vi "Constructor.vi"(8 "error in (no error)":errorcluster, 11 "Reference":refnum<vi>) -> (0 "error out":errorcluster, 3 "MCLB":refnum<class "Selector.lvclass">)   [LabVIEW 2019, in "Selector.lvclass"]
uses:
  Selector.lvclass
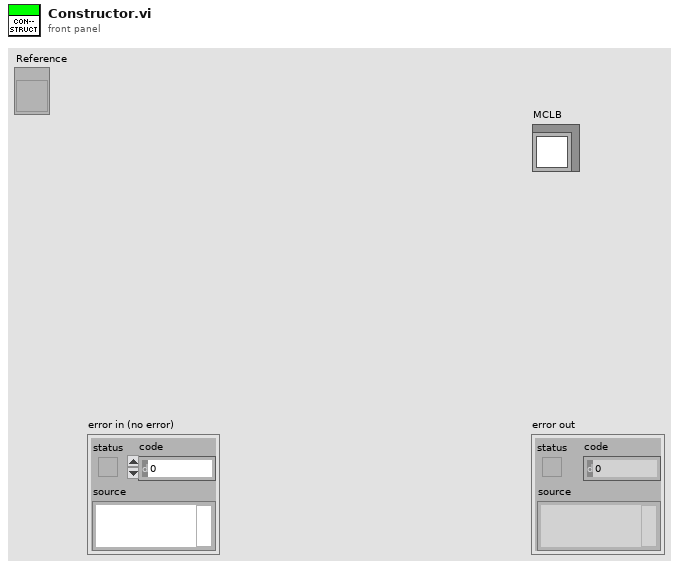
[diagram p1: front panel]
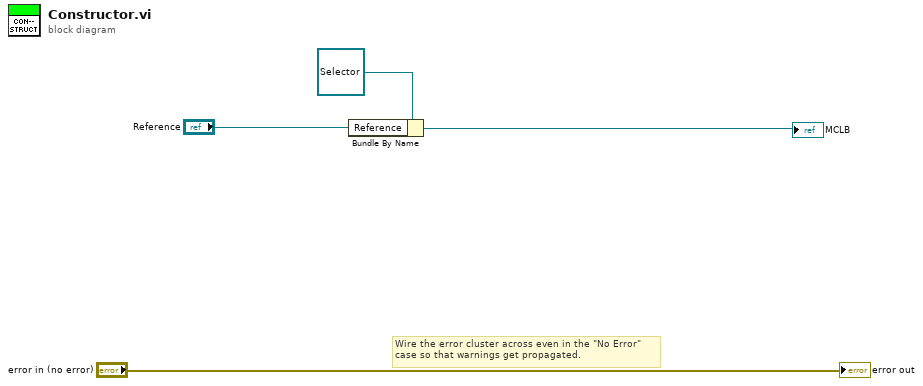
[diagram p0: block diagram]
diagram:
  # "Wire the error cluster across even in the \"No Error\"\ncase so that warnings get propagated."
  n1 = Bundle By Name(cluster=refnum<class "Selector.lvclass"> refnum ("Selector out"), "Reference"="Reference") -> (→"MCLB":refnum<class "Selector.lvclass">)
  "error out" <- "error in (no error)"
